vi "AssembleVelocityStats.vi"(7 "TitlePrefix":string, 11 "VmagUVWCone":dbl[][](array[numeric])) -> (1 "Plug in titles":string[](array[string]), 3 "StatsArray":dbl[](array[numeric]))   [LabVIEW 2016]
uses:
  <vilib>/Analysis/NI_AALBase.lvlib
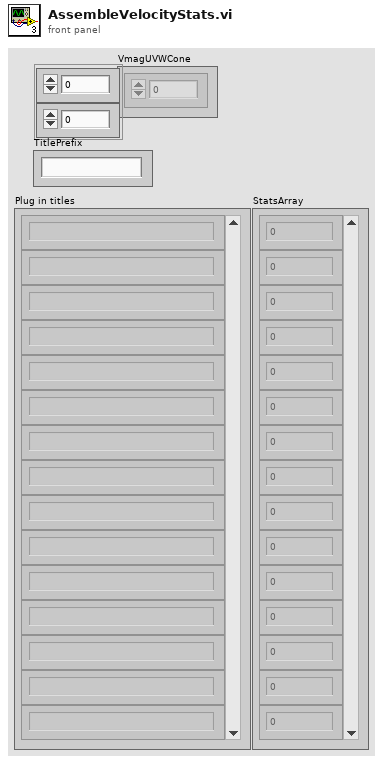
[diagram p1: front panel]
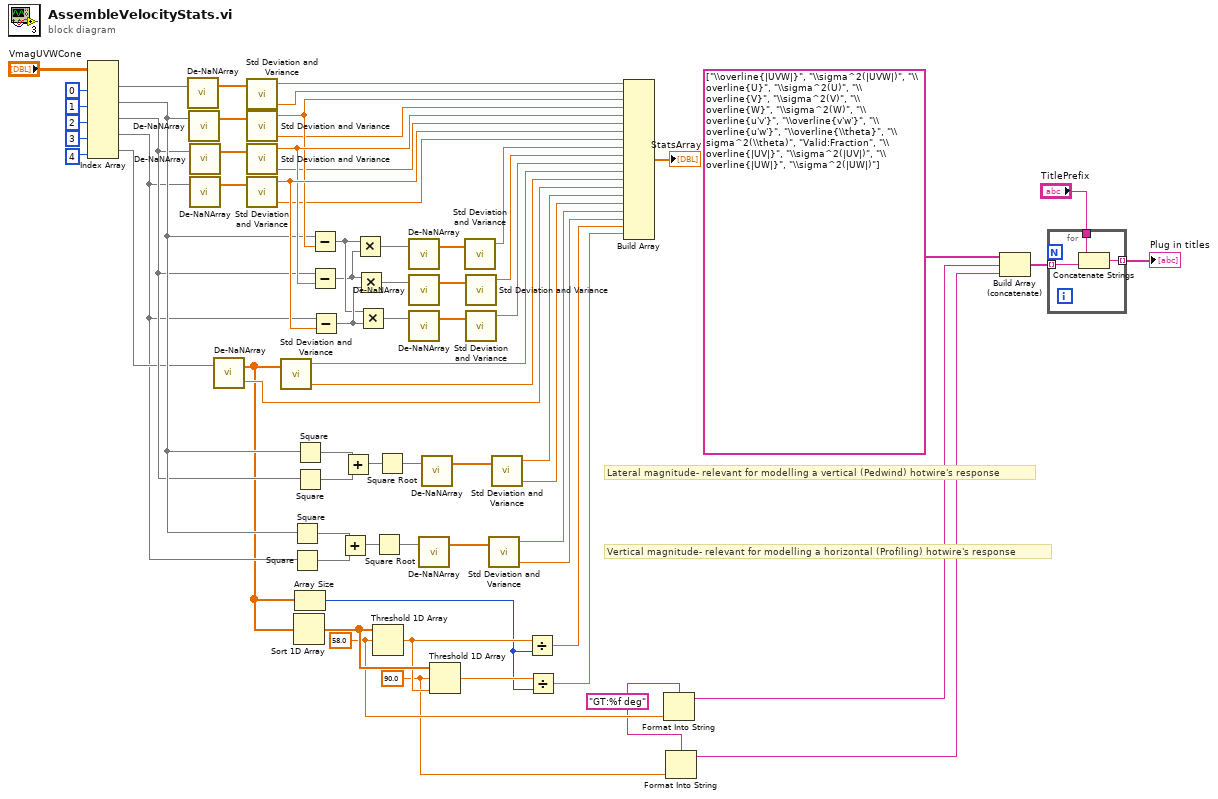
[diagram p0: block diagram]
diagram:
  w4 = "GT:%f deg" ("format string")
  w5 = 90.0 ("threshold y")
  w6 = 58.0 ("threshold y")
  # "Vertical magnitude- relevant for modelling a horizontal (Profiling) hotwire's response"
  # "Lateral magnitude- relevant for modelling a vertical (Pedwind) hotwire's response"
  n1 = Index Array(array="VmagUVWCone", index (col) #1=0 ("disabled index (col)"), index (col) #2=1 ("index (col)"), index (col) #3=2 ("index (col)"), index (col) #4=3 ("index (col)"), index (col) #5=4 ("index (col)")) -> (element #1=w19:dbl[], element #2=w17:dbl[], element #3=w16:dbl[], element #4=w14:dbl[], element #5=w15:dbl[])  [unwired: 5 in]
  n2 = call "De-NaNArray.vi"("ArrayIn"=w19) -> ("de-NaN-dArrayOut"=w34:dbl[])  [unwired: 1 in, 1 out]
  n3 = call "De-NaNArray.vi"("ArrayIn"=w17) -> ("de-NaN-dArrayOut"=w43:dbl[])  [unwired: 1 in, 1 out]
  n4 = call "De-NaNArray.vi"("ArrayIn"=w16) -> ("de-NaN-dArrayOut"=w42:dbl[])  [unwired: 1 in, 1 out]
  n5 = call "De-NaNArray.vi"("ArrayIn"=w14) -> ("de-NaN-dArrayOut"=w41:dbl[])  [unwired: 1 in, 1 out]
  n6 = call "De-NaNArray.vi"("ArrayIn"=w15) -> ("GoodFraction"=w33:dbl, "de-NaN-dArrayOut"=w12:dbl[])  [unwired: 1 in]
  n7 = call <vilib>:"Std Deviation and Variance.vi"("X"=w34) -> ("mean"=w57:dbl, "variance"=w52:dbl)  [unwired: 1 in, 1 out]
  n8 = call <vilib>:"Std Deviation and Variance.vi"("X"=w43) -> ("mean"=w58:dbl, "variance"=w53:dbl)  [unwired: 1 in, 1 out]
  n9 = call <vilib>:"Std Deviation and Variance.vi"("X"=w42) -> ("mean"=w59:dbl, "variance"=w54:dbl)  [unwired: 1 in, 1 out]
  n10 = call <vilib>:"Std Deviation and Variance.vi"("X"=w41) -> ("mean"=w60:dbl, "variance"=w55:dbl)  [unwired: 1 in, 1 out]
  n11 = call <vilib>:"Std Deviation and Variance.vi"("X"=w12) -> ("mean"=w68:dbl, "variance"=w69:dbl)  [unwired: 1 in, 1 out]
  n12 = Square(x=w17) -> (x^2=w22:dbl[])
  n13 = Square(x=w14) -> (x^2=w23:dbl[])
  n14 = Sort 1D Array(array=w12) -> (sorted array=w13:dbl[])
  n15 = Square(x=w17) -> (x^2=w32:dbl[])
  n16 = Square(x=w16) -> (x^2=w31:dbl[])
  n17 = Array Size(array=w12) -> (size(s)=w9:i32)
  n18 = Subtract(x=w17, y=w58) -> (x-y=w62:dbl[])
  n19 = Subtract(x=w16, y=w59) -> (x-y=w61:dbl[])
  n20 = Subtract(x=w14, y=w60) -> (x-y=w63:dbl[])
  n21 = Add(x=w22, y=w23) -> (x+y=w24:dbl[])
  n22 = Add(x=w32, y=w31) -> (x+y=w30:dbl[])
  n23 = Multiply(x=w62, y=w61) -> (x*y=w40:dbl[])
  n24 = Multiply(x=w61, y=w63) -> (x*y=w38:dbl[])
  n25 = Multiply(x=w62, y=w63) -> (x*y=w36:dbl[])
  n26 = Threshold 1D Array(2:w6, 3:w13) -> (0:w11:dbl)  [unwired: 1 in]
  n27 = Square Root(x=w24) -> (sqrt(x)=w25:dbl[])
  n28 = Square Root(x=w30) -> (sqrt(x)=w18:dbl[])
  n29 = call "De-NaNArray.vi"("ArrayIn"=w40) -> ("de-NaN-dArrayOut"=w39:dbl[])  [unwired: 1 in, 1 out]
  n30 = call "De-NaNArray.vi"("ArrayIn"=w38) -> ("de-NaN-dArrayOut"=w37:dbl[])  [unwired: 1 in, 1 out]
  n31 = call "De-NaNArray.vi"("ArrayIn"=w36) -> ("de-NaN-dArrayOut"=w35:dbl[])  [unwired: 1 in, 1 out]
  n32 = call "De-NaNArray.vi"("ArrayIn"=w25) -> ("de-NaN-dArrayOut"=w26:dbl[])  [unwired: 1 in, 1 out]
  n33 = call "De-NaNArray.vi"("ArrayIn"=w18) -> ("de-NaN-dArrayOut"=w29:dbl[])  [unwired: 1 in, 1 out]
  n34 = Threshold 1D Array(1:w11, 2:w5, 3:w13) -> (0:w10:dbl)
  n35 = call <vilib>:"Std Deviation and Variance.vi"("X"=w39) -> ("mean"=w64:dbl)  [unwired: 1 in, 2 out]
  n36 = call <vilib>:"Std Deviation and Variance.vi"("X"=w37) -> ("mean"=w65:dbl)  [unwired: 1 in, 2 out]
  n37 = call <vilib>:"Std Deviation and Variance.vi"("X"=w35) -> ("mean"=w66:dbl)  [unwired: 1 in, 2 out]
  n38 = call <vilib>:"Std Deviation and Variance.vi"("X"=w26) -> ("mean"=w21:dbl, "variance"=w20:dbl)  [unwired: 1 in, 1 out]
  n39 = call <vilib>:"Std Deviation and Variance.vi"("X"=w29) -> ("mean"=w28:dbl, "variance"=w27:dbl)  [unwired: 1 in, 1 out]
  n40 = Divide(x=w11, y=w9) -> (x/y=w8:dbl)
  n41 = Divide(x=w10, y=w9) -> (x/y=w7:dbl)
  n42 = Build Array(w57, w52, w58, w53, w59, w54, w60, w55, w64, w65, w66, w68, w69, w33, w28, w27, w21, w20, w8, w7) -> (→"StatsArray":dbl[])
  n43 = Format Into String(format string=w4, w6) -> (resulting string=w2:string)  [unwired: 2 in, 1 out]
  n44 = Format Into String(format string=w4, w5) -> (resulting string=w1:string)  [unwired: 2 in, 1 out]
  n45 = Build Array (concatenate)(string[] ["\\overline{|UVW|}", "\\sigma^2(|UVW|)", "\\overline{U}", "\\sigma^2(U)", "\\overline{V}", "\\sigma^2(V)", "\\overline{W}", "\\sigma^2(W)", "\\overline{u'v'}", "\\overline{v'w'}", "\\overline{u'w'}", "\\overline{\\theta}", "\\sigma^2(\\theta)", "Valid:Fraction", "\\overline{|UV|}", "\\sigma^2(|UV|)", "\\overline{|UW|}", "\\sigma^2(|UW|)"] ("Plug in titles"), w2, w1) -> (w3:string[])
  n46 = for {
    tunnel: w3 -> [w72] mode=indexing
    tunnel: "TitlePrefix" -> [w71]
    tunnel: [w70] -> w44 mode=indexing
    n47 = Concatenate Strings(w71, w72) -> (w70:string)
  }
  "Plug in titles" <- w44
